vi "check focus or flystart.vi"(11 "GFG variable name":string) -> (3 "Focus or flystart?":bool)   [LabVIEW 2017]
doc: "SciScan 1.2 160622"
uses:
  GFG/GFGbooleanGet.vi
  GFG/GFG library.lvlib
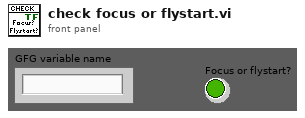
[diagram p1: front panel]
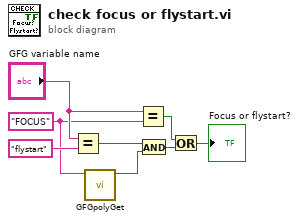
[diagram p0: block diagram]
diagram:
  w1 = "FOCUS" ("y")
  n1 = Equal?(x="GFG variable name", y="flystart") -> (x = y?=w6:bool)
  n2 = call-poly "GFGpolyGet.vi"("Variable Name in"=w1) -> ("Boolean Value OUT"=w4:bool)  [unwired: 9 in, 1 out]
  n3 = Equal?(x="GFG variable name", y=w1) -> (x = y?=w8:bool)
  n4 = And(x=w6, y=w4) -> (x .and. y?=w5:bool)
  n5 = Or(x=w8, y=w5) -> (x .or. y?=→"Focus or flystart?":bool)
